vi "DFD Integer Delay (Wfm NChan).vi"(7 "init? (F)":bool, 8 "error in (no error)":errorcluster, 10 "delay":i32, 11 "signal in":waveform(dbl)[](array[waveform])) -> (0 "error out":errorcluster, 3 "signal out":waveform(dbl)[](array[waveform]))   [LabVIEW 2017, in "NI_DigFilterLicensed.lvlib"]
doc: "Delays a signal continuously by a specified integer number of sample intervals. Wire data to the <B>signal in</B> input to determine the polymorphic instance to use or manually select the instance."
uses:
  <vilib>/addons/Digital Filter Design/NI_DigFilterLicensed.lvlib
  <vilib>/addons/Digital Filter Design/Process.llb/DFD Integer Delay with State (Array).vi
  <vilib>/addons/Digital Filter Design/NI_DigFilter_Process.lvlib
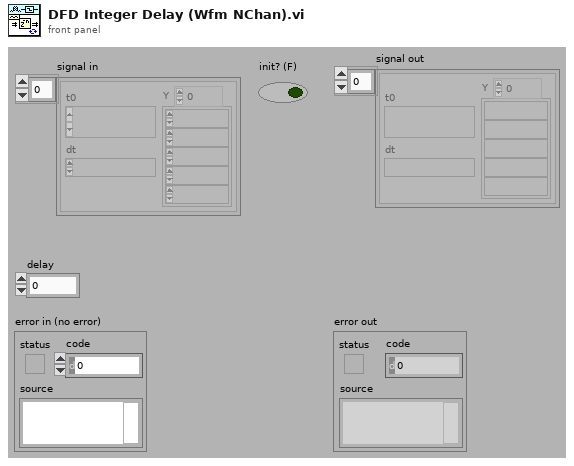
[diagram p1: front panel]
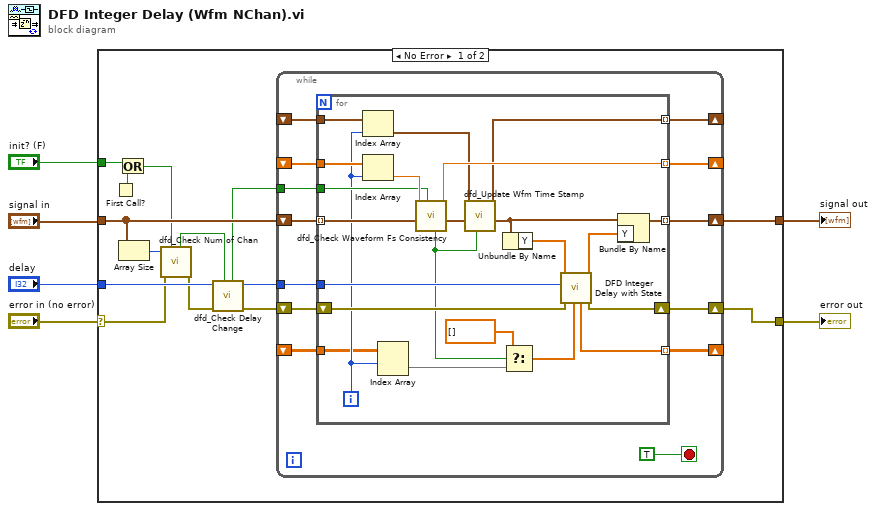
[diagram p0: block diagram]
diagram:
  n1 = case shown="No Error" "error in (no error)" {
    selector: "error in (no error)" -> [w11 w57]
    tunnel: [w19 w57] -> w3
    tunnel: "signal in" -> [w16 _]
    tunnel: [w20 _] -> w5
    tunnel: "delay" -> [w13 _]
    tunnel: "init? (F)" -> [w17 _]
    frame No Error {
      n2 = First Call?() -> (First Call?: T/F=w18:bool)
      n3 = Or(x=w17, y=w18) -> (x .or. y?=w14:bool)
      n4 = Array Size(array=w16) -> (size(s)=w15:i32)
      n5 = call <vilib>:"dfd_Check Num of Chan.vi"("init in"=w14, "error in (no error)"=w11, "#ch in"=w15) -> ("error out"=w10:errorcluster, "init out"=w12:bool)  [unwired: 7 out]
      n6 = call <vilib>:"dfd_Check Delay Change.vi"("init in"=w12, "error in (no error)"=w10, "delay in"=w13) -> ("error out"=w9:errorcluster, "delay out"=w7:i32, "init out"=w8:bool)  [unwired: 6 out]
      n7 = while {
        shift-right: [w30] -> _
        shift-left: _ -> [w21]
        tunnel: w7 -> [w28]
        shift-right: [w32] -> w20
        shift-left: w16 -> [w33]
        shift-right: [w27] -> w19
        shift-left: w9 -> [w29]
        shift-right: [w25] -> _
        shift-left: _ -> [w26]
        shift-right: [w22] -> _
        shift-left: _ -> [w24]
        tunnel: w8 -> [w23]
        stop <- TRUE stop-if-true
        n8 = for {
          tunnel: w33 -> [w56] mode=indexing
          tunnel: [w45] -> w32 mode=indexing
          tunnel: [w38] -> w30 mode=indexing
          tunnel: w28 -> [w43]
          shift-right: [w41] -> w27
          shift-left: w29 -> [w42]
          tunnel: w26 -> [w55]
          tunnel: [w54] -> w25 mode=indexing
          tunnel: w24 -> [w52]
          tunnel: w23 -> [w50]
          tunnel: [w48] -> w22 mode=indexing
          tunnel: w21 -> [w39]
          i -> [w40]
          n9 = Index Array(array=w52, index=w40) -> (element=w49:timestamp)
          n10 = Index Array(array=w55, index=w40) -> (element=w53:dbl)
          n11 = Index Array(array=w39, index (row)=w40) -> (element=w37:dbl[])  [unwired: 1 in]
          n12 = call <vilib>:"dfd_Check Waveform Fs Consistency.vi"("init in"=w50, "signal in"=w56, "dt in"=w53) -> ("signal out"=w51:waveform(dbl), "dt out"=w54:dbl, "init out"=w34:bool)  [unwired: 1 in, 5 out]
          n13 = call <vilib>:"dfd_Update Wfm Time Stamp.vi"("init? (F)"=w34, "signal in"=w51, "t0"=w49) -> ("signal out"=w46:waveform(dbl), "tf"=w48:timestamp)  [unwired: 7 out]
          n14 = Unbundle By Name(w46) -> ("Y"=w47:dbl[])
          n15 = Select(t=dbl[] [], s=w34, f=w37) -> (s? t:f=w36:dbl[])
          n16 = call-poly <vilib>:"DFD Integer Delay with State.vi"("state in"=w36, "error in (no error)"=w42, "delay"=w43, "signal in"=w47) -> ("error out"=w41:errorcluster, "signal out"=w44:dbl[], "state out"=w38:dbl[])  [unwired: 5 out]
          n17 = Bundle By Name(cluster=w46, "Y"=w44) -> (w45:waveform(dbl))
        }
      }
    }
    frame Error {
    }
  }
  "error out" <- w3
  "signal out" <- w5
